vi "Teardown.vi"(8 "error in (no error)":errorcluster, 11 "Coverage Report Test In":refnum<class "Coverage Report Test.lvclass">) -> (0 "error out":errorcluster, 3 "Coverage Report Test Out":refnum<class "Coverage Report Test.lvclass">)   [LabVIEW 2020, in "Coverage Report Test.lvclass"]
doc: "Teardown method called by the testing framework to tear down test fixture after each test method is called."
uses:
  Coverage Report Test.lvclass
  Coverage Report Test.lvclass/Coverage Report Test.ctl
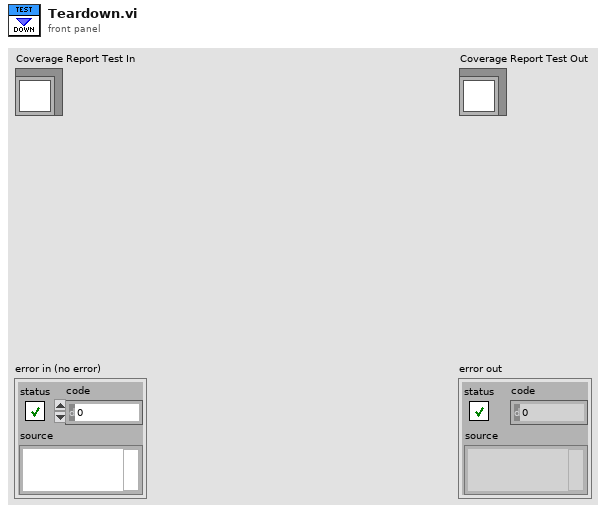
[diagram p1: front panel]
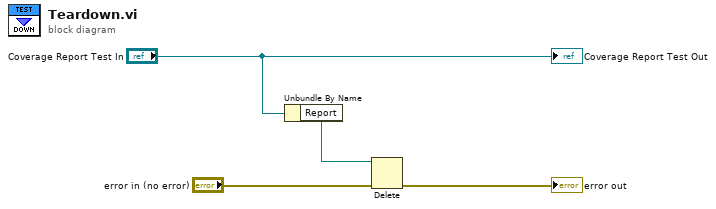
[diagram p0: block diagram]
diagram:
  n1 = Unbundle By Name("Coverage Report Test In") -> ("Report"=w1:path)
  n2 = Delete(path (use dialog)=w1, error in="error in (no error)") -> (error out=→"error out":errorcluster)  [unwired: 3 in, 2 out]
  "Coverage Report Test Out" <- "Coverage Report Test In"
